vi "DynamicLoadMemoryMap.vi"(7 "ApplicationPath":path, 8 "error in (no error)":errorcluster, 11 "Gserver in":refnum<class "Gserver.lvclass">) -> (0 "error out":errorcluster, 3 "Gserver out":refnum<class "Gserver.lvclass">)   [LabVIEW 2020, in "Gserver.lvclass"]
doc: "Andre Koelewijn, 2 jan 2021\n\nDynamically open a new Gviewer application instance.\nThe name of the new instance depends upon the numbers of open graphs and is determined by Gserver.\nThe maximum number of allowed graphs is defined as provided to this vi."
uses:
  Gserver.lvclass
  Gserver.lvclass/Gserver.ctl
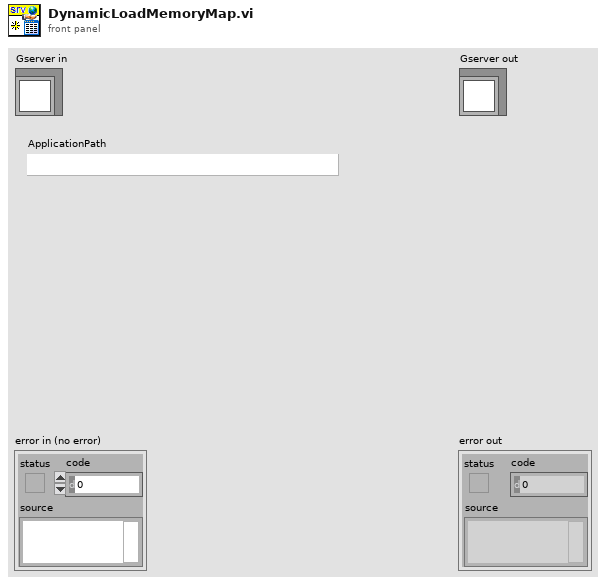
[diagram p1: front panel]
types:
  T1 = enum32{"Invalid", "Standard", "Closed", "Hidden", "Minimized", "Maximized"}
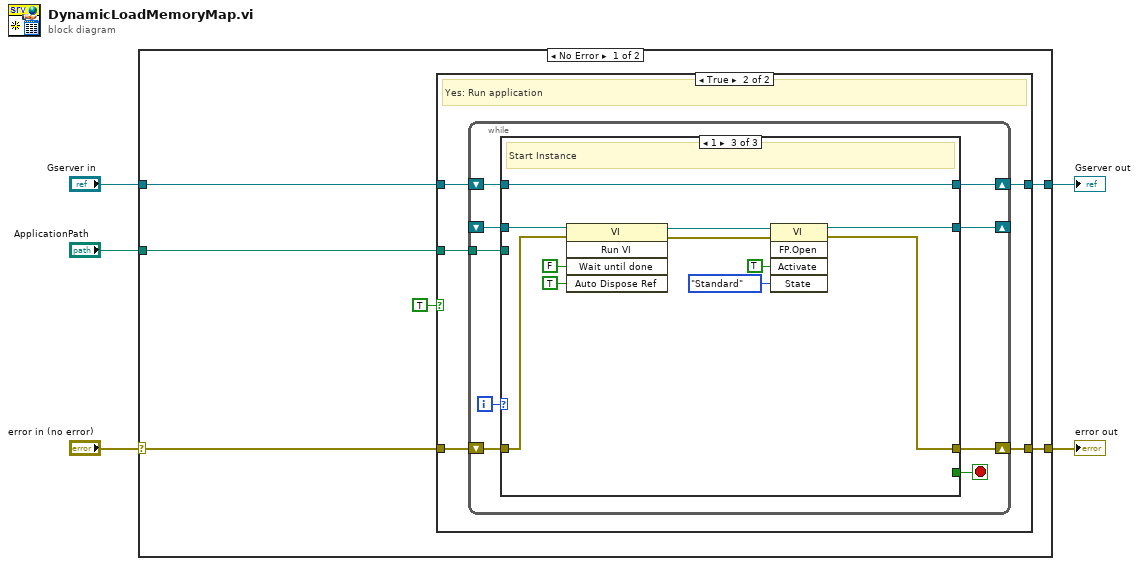
[diagram p0: block diagram]
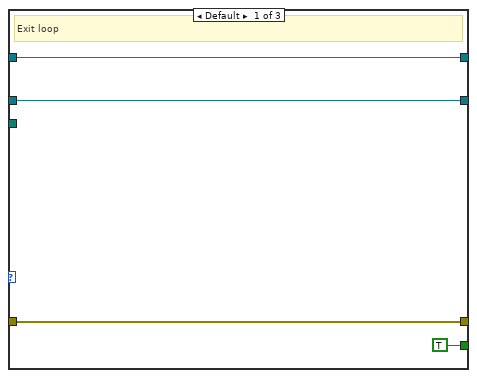
[diagram p3: hidden frame]
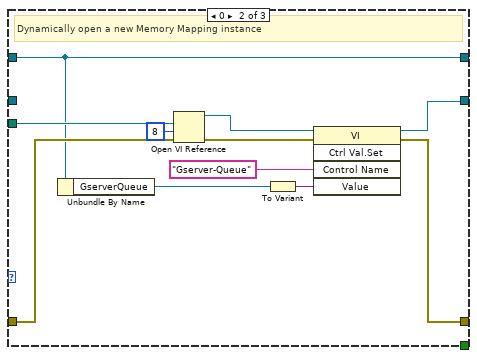
[diagram p4: hidden frame]
diagram:
  n1 = case shown="No Error" "error in (no error)" {
    selector: "error in (no error)" -> [w10 w55]
    tunnel: [w7 w55] -> w4
    tunnel: [w9 w54] -> w2
    tunnel: "Gserver in" -> [w8 w54]
    tunnel: "ApplicationPath" -> [w11 _]
    frame No Error {
      n2 = case shown="True" TRUE {
        tunnel: w11 -> [_ w18]
        tunnel: w10 -> [w12 w17]
        tunnel: [w13 w16] -> w9
        tunnel: w8 -> [w13 w15]
        tunnel: [w12 w14] -> w7
        frame False {
          # "Do not start if already running"
        }
        frame True {
          # "Yes: Run application"
          n3 = while {
            tunnel: w18 -> [w27]
            shift-right: [w23] -> w16
            shift-left: w15 -> [w24]
            shift-right: [w21] -> w14
            shift-left: w17 -> [w26]
            shift-right: [w22] -> _
            shift-left: _ -> [w20]
            i -> [w25]
            stop <- w19 stop-if-true
            n4 = case shown="1" w25 {
              tunnel: w27 -> [_ w42 _]
              tunnel: w26 -> [w29 w41 w44]
              tunnel: w24 -> [w30 w38 w53]
              tunnel: [w30 w38 w53] -> w23
              tunnel: [w31 w33 w47] -> w22
              tunnel: [w29 w34 w45] -> w21
              tunnel: w20 -> [w31 _ w52]
              tunnel: [TRUE _ _] -> w19
              frame Default {
                # "Exit loop"
              }
              frame 0 {
                # "Dynamically open a new Memory Mapping instance"
                n5 = Unbundle By Name(w38) -> ("GserverQueue"=w37:refnum<queue>)
                n6 = Open VI Reference(vi path=w42, options=8, error in (no error)=w41) -> (vi reference=w39:refnum<vi>, error out=w35:errorcluster)  [unwired: 3 in]
                n7 = To Variant(anything=w37) -> (Variant=w36:variant)
                n8 = invoke class="VI" method="Ctrl Val.Set"(reference=w39, error in=w35, "Control Name"="Gserver-Queue", "Value"=w36) -> (reference out=w33:refnum<vi>, error out=w34:errorcluster)  [unwired: 1 in, 3 out]
              }
              frame 1 {
                # "Start Instance"
                n9 = invoke class="VI" method="Run VI"(reference=w52, error in=w44, "Wait until done"=FALSE ("Wait Until Done"), "Auto Dispose Ref"=TRUE ("Auto Dispose Reference")) -> (reference out=w48:refnum<vi>, error out=w46:errorcluster)  [unwired: 1 in, 3 out]
                n10 = invoke class="VI" method="FP.Open"(reference=w48, error in=w46, "Activate"=TRUE ("Wait Until Done"), "State"=T1."Standard") -> (reference out=w47:refnum<vi>, error out=w45:errorcluster)  [unwired: 1 in, 3 out]
              }
            }
          }
        }
      }
    }
    frame Error {
    }
  }
  "error out" <- w4
  "Gserver out" <- w2
